vi "LogQuickNote.vi"(8 "error in (no error)":errorcluster, 10 "New Image":T1, 11 "DataLogger in":refnum<class "DataLogger.lvclass">) -> (0 "error out":errorcluster, 2 "Image Out":T1, 3 "DataLogger out":refnum<class "DataLogger.lvclass">)   [LabVIEW 2020, in "DataLogger.lvlib" / "DataLogger.lvclass"]
uses:
  DataLogger.lvclass
  <vilib>/vision/Image Controls.llb/IMAQ Image.ctl
  DataLogger.lvclass/DataLogger.ctl
panel:
  out "Keys":string[](array[string])
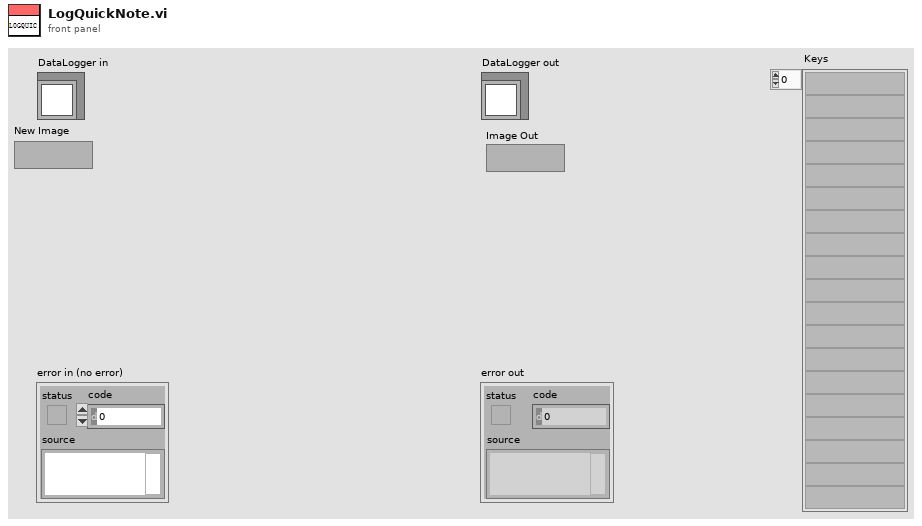
[diagram p1: front panel]
types:
  T1 = typedef "IMAQ Image.ctl" = refnum<image>
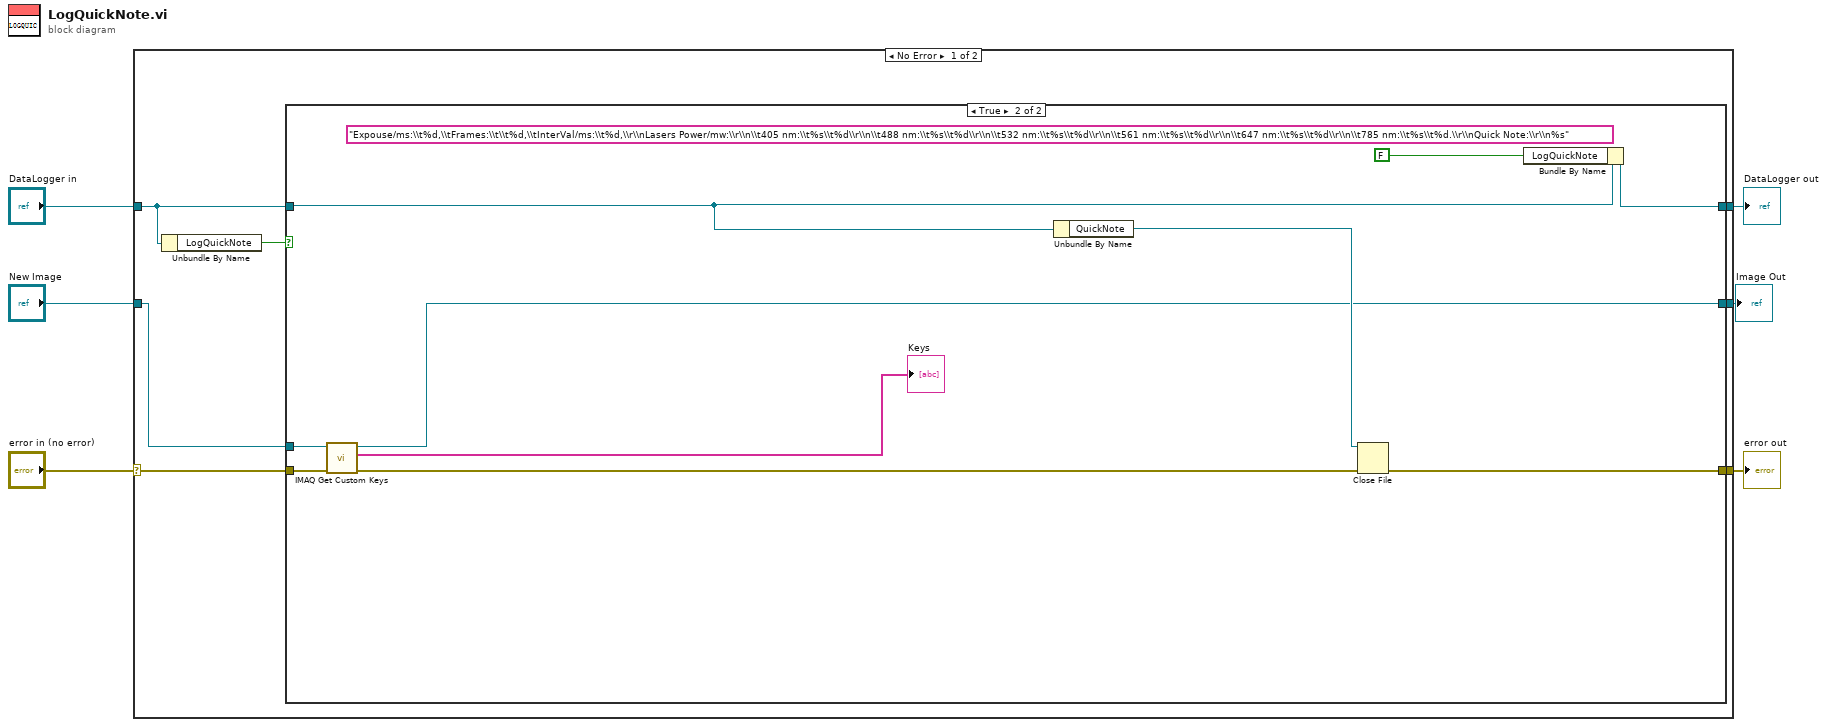
[diagram p0: block diagram]
diagram:
  n1 = case shown="No Error" "error in (no error)" {
    selector: "error in (no error)" -> [w13 w29]
    tunnel: [w10 w29] -> w5
    tunnel: [w9 w28] -> w3
    tunnel: "DataLogger in" -> [w8 w28]
    tunnel: "New Image" -> [w12 w27]
    tunnel: [w11 w27] -> w1
    frame No Error {
      n2 = Unbundle By Name(w8) -> ("LogQuickNote"=w7:bool)
      n3 = case shown="True" w7 {
        tunnel: w13 -> [w15 w26]
        tunnel: w12 -> [w14 w19]
        tunnel: [w14 w18] -> w11
        tunnel: [w15 w21] -> w10
        tunnel: w8 -> [w16 w23]
        tunnel: [w16 w25] -> w9
        frame False {
        }
        frame True {
          (unwired) "Expouse/ms:\\t%d,\\tFrames:\\t\\t%d,\\tInterVal/ms:\\t%d,\\r\\nLasers Power/mw:\\r\\n\\t405 nm:\\t%s\\t%d\\r\\n\\t488 nm:\\t%s\\t%d\\r\\n\\t532 nm:\\t%s\\t%d\\r\\n\\t561 nm:\\t%s\\t%d\\r\\n\\t647 nm:\\t%s\\t%d\\r\\n\\t785 nm:\\t%s\\t%d.\\r\\nQuick Note:\\r\\n%s" ("format string")
          n4 = call "IMAQ Get Custom Keys"("error in (no error)"=w26, "Image"=w19) -> ("error out"=w20:errorcluster, "Keys"=→"Keys":string[], "Image (duplicate)"=w18:T1)  [unwired: 6 in, 1 out]
          n5 = Unbundle By Name(w23) -> ("QuickNote"=w22:refnum<file>)
          n6 = Close File(refnum=w22, error in=w20) -> (error out=w21:errorcluster)  [unwired: 1 out]
          n7 = Bundle By Name(cluster=w23, "LogQuickNote"=FALSE) -> (w25:refnum<class "DataLogger.lvclass">)
        }
      }
    }
    frame Error {
    }
  }
  "error out" <- w5
  "DataLogger out" <- w3
  "Image Out" <- w1
